vi "ex_convert2DArrayToExWave.vi"(6 "Origin Timestamp":timestamp format="%<%X\n%x>T", 8 "error in (no error)":errorcluster, 9 "Relative Time?":bool, 10 "channel info":T1[](array[typedef]) {"Delta X" format="%.2p"; "X0" format="%<%X\n%x>T"; "Timestamp" format="%<%X\n%x>T"}, 11 "Y Data":dbl[][](array[numeric]) format="%0.2f") -> (0 "error out":errorcluster, 2 "Express Attributes":T2[](array[typedef]) {"dX" format="%.2f"; "X0" format="%<%X\n%x>T"; "Timestamp" format="%<%X\n%x>T"; "Start Timestamp" format="%<%X\n%x>T"}, 3 "Signals":waveform(dbl)[](array[waveform]))   [LabVIEW 2020]
uses:
  <vilib>/express/express shared/transition.llb/ex_WaveformAttribsPlus.ctl
  <vilib>/express/express shared/ExFile.llb/ex_AllChanInfo.ctl
panel:
  in  "Express Attributes":T2 {"dX" format="%.2f"; "X0" format="%<%X\n%x>T"; "Timestamp" format="%<%X\n%x>T"; "Start Timestamp" format="%<%X\n%x>T"}
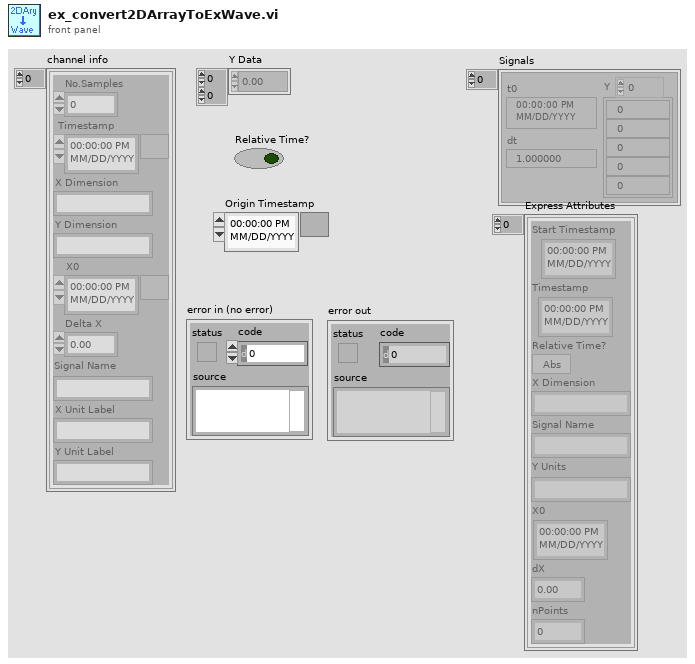
[diagram p1: front panel]
types:
  T1 = typedef "ex_AllChanInfo.ctl" = cluster{"No.Samples":i32, "Timestamp":timestamp, "X Dimension":string, "Y Dimension":string, "X0":timestamp, "Delta X":dbl, "Signal Name":string, "X Unit Label":string, "Y Unit Label":string}
  T2 = typedef "ex_WaveformAttribsPlus.ctl" = cluster{"Start Timestamp":timestamp, "Timestamp":timestamp, "Relative Time?":bool, "X Dimension":string, "Signal Name":string, "Y Units":string, "X0":timestamp, "dX":dbl, "nPoints":i32}
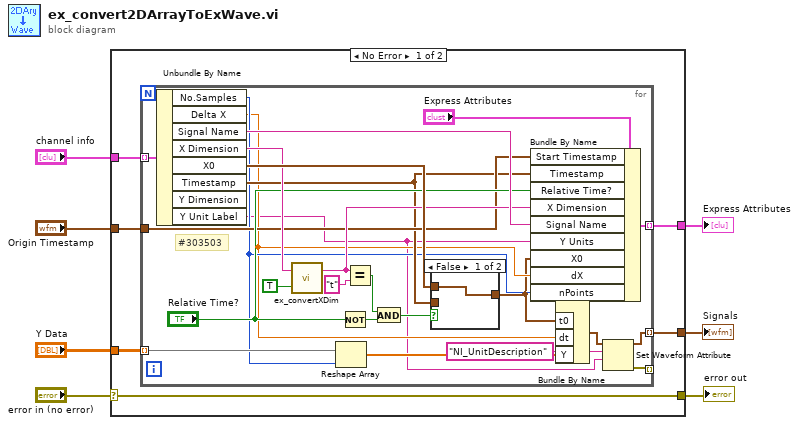
[diagram p0: block diagram]
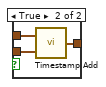
[diagram p2: hidden frame]
diagram:
  n1 = case shown="No Error" "error in (no error)" {
    selector: "error in (no error)" -> [w8 w43]
    tunnel: [w13 _] -> w7
    tunnel: "Origin Timestamp" -> [w12 _]
    tunnel: [w11 _] -> w5
    tunnel: "Y Data" -> [w10 _]
    tunnel: "channel info" -> [w9 _]
    tunnel: [w8 w43] -> w1
    frame No Error {
      n2 = for {
        tunnel: w9 -> [w38] mode=indexing
        tunnel: w10 -> [w37] mode=indexing
        tunnel: [w17] -> w13 mode=indexing
        tunnel: [w32] -> w11 mode=indexing
        tunnel: w12 -> [w24]
        tunnel: [w16] -> _ mode=indexing
        # "#303503"
        n3 = Unbundle By Name(w38) -> ("No.Samples"=w22:i32, "Delta X"=w21:dbl, "Signal Name"=w33:string, "X Dimension"=w30:string, "X0"=w34:timestamp, "Timestamp"=w23:timestamp, "Y Unit Label"=w14:string)  [unwired: 1 out]
        n4 = call <vilib>:"ex_convertXDim.vi"("mode (F:Code to String)"=TRUE, "x_dimension in"=w30) -> ("x_dimension out"=w29:string)  [unwired: 1 out]
        n5 = Reshape Array(w37, w22) -> (w36:dbl[])
        n6 = Not(x="Relative Time?") -> (.not. x?=w26:bool)
        n7 = Equal?(x=w29, y="t") -> (x = y?=w25:bool)
        n8 = And(x=w25, y=w26) -> (x .and. y?=w19:bool)
        n9 = case shown="False" w19 {
          tunnel: w34 -> [w39 w42]
          tunnel: w23 -> [_ w41]
          tunnel: [w39 w40] -> w20
          frame False {
          }
          frame True {
            n10 = call <vilib>:"Timestamp Add.vi"("y"=w41, "x"=w42) -> ("x + y"=w40:timestamp)
          }
        }
        n11 = Bundle By Name(cluster="Express Attributes", "Start Timestamp"=w24, "Timestamp"=w23, "Relative Time?"="Relative Time?", "X Dimension"=w29, "Signal Name"=w33, "Y Units"=w14, "X0"=w20, "dX"=w21, "nPoints"=w22) -> (w32:T2)
        n12 = Bundle By Name("t0"=w20, "dt"=w21, "Y"=w36) -> (w18:waveform(dbl))  [unwired: 1 out]
        n13 = Set Waveform Attribute(5:w14, 6:"NI_UnitDescription" ("name"), 7:w18) -> (0:w16:errorcluster, 3:w17:waveform(dbl))  [unwired: 1 in, 1 out]
      }
    }
    frame Error {
    }
  }
  "Signals" <- w7
  "Express Attributes" <- w5
  "error out" <- w1
